vi "RT Driver VI.vi"(7 "Operation":T1, 11 "Device Reference in":T2 format="%.0x") -> (0 "Error Code":i32)   [LabVIEW 2019, in "Inline Telemetry Prototype Engine.lvlib"]
uses:
  Inline Telemetry Prototype Engine.lvlib
  <vilib>/NI VeriStand/Custom Device API/Custom Device Item Ref.ctl
  <vilib>/NI VeriStand/Custom Device API/Hardware Interface Driver VI Operation.ctl
  <vilib>/NI VeriStand/Custom Device API/Data Access Type.ctl
  Inline Async CD Template/Engine/Loop Data.ctl
  <vilib>/NI VeriStand/Custom Device API/Block Data Reference.ctl
  <vilib>/NI VeriStand/Custom Device API/Data Reference.ctl
  <vilib>/NI VeriStand/Custom Device API/Global Data Refs.vi
  <vilib>/NI VeriStand/Custom Device API/Custom Device API.lvlib
  Inline Async CD Template/Engine/Inline Async CD Template Engine.lvlib
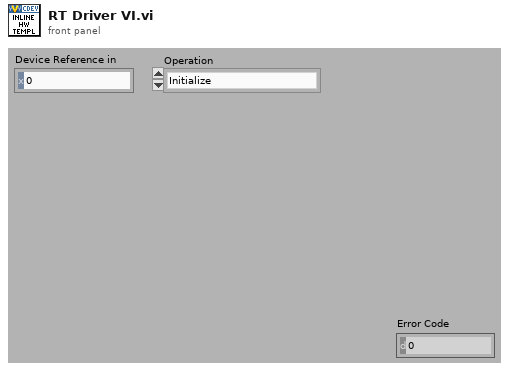
[diagram p1: front panel]
types:
  T1 = typedef "Custom Device API.lvlib/Hardware Interface Driver VI Operation.ctl" = enum16{"Initialize", "Start", "Read Data from HW", "Write Data to HW", "Close"}
  T2 = typedef "Custom Device API.lvlib/Custom Device Item Ref.ctl" = u64
  T3 = typedef "Inline Async CD Template Engine.lvlib/Loop Data.ctl" = cluster{"Device Error":errorcluster, "Data FIFO":refnum<k33>, "Block Data Refs":T4[], "Data":dbl[]}
  T4 = typedef "Custom Device API.lvlib/Block Data Reference.ctl" = cluster{"Data Reference":T5, "Offset":u64, "Length":u64}
  T5 = typedef "Custom Device API.lvlib/Data Reference.ctl" = i32
  T6 = typedef "Custom Device API.lvlib/Data Access Type.ctl" = enum16{"Read", "Write"}
  T7 = cluster{"read mode":enum16{"polling", "blocking"}, "write mode":enum16{"polling", "blocking"}}
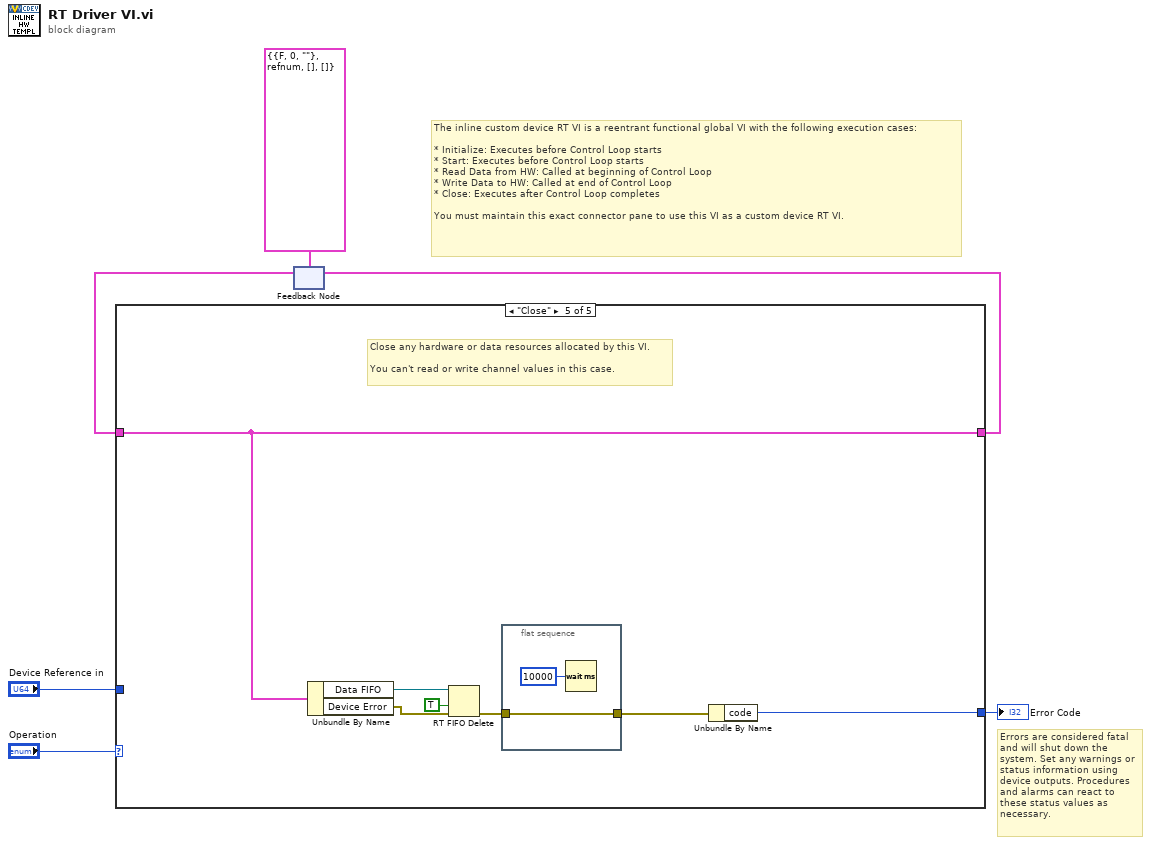
[diagram p0: block diagram]
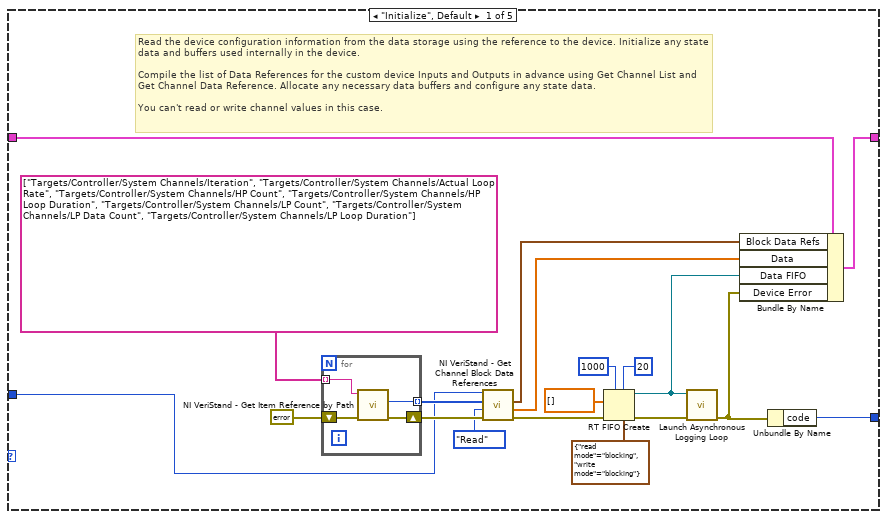
[diagram p2: hidden frame]
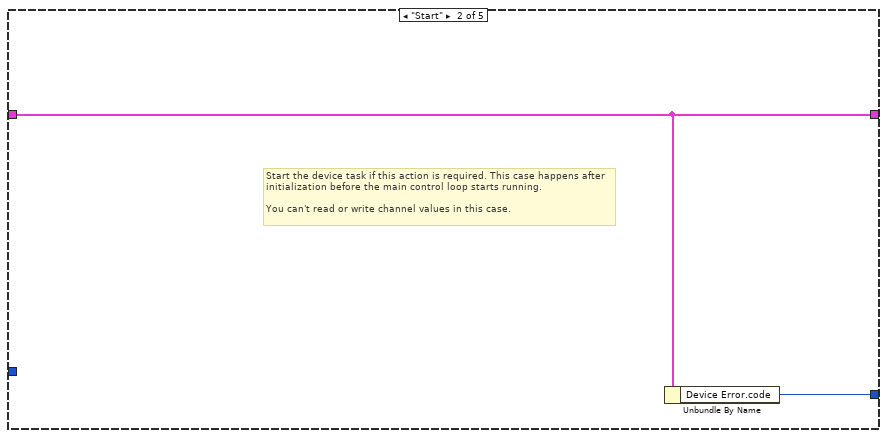
[diagram p3: hidden frame]
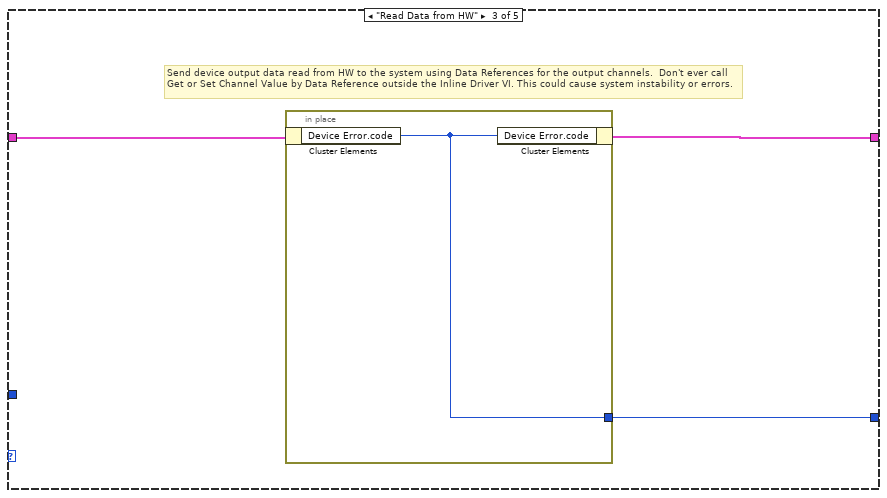
[diagram p4: hidden frame]
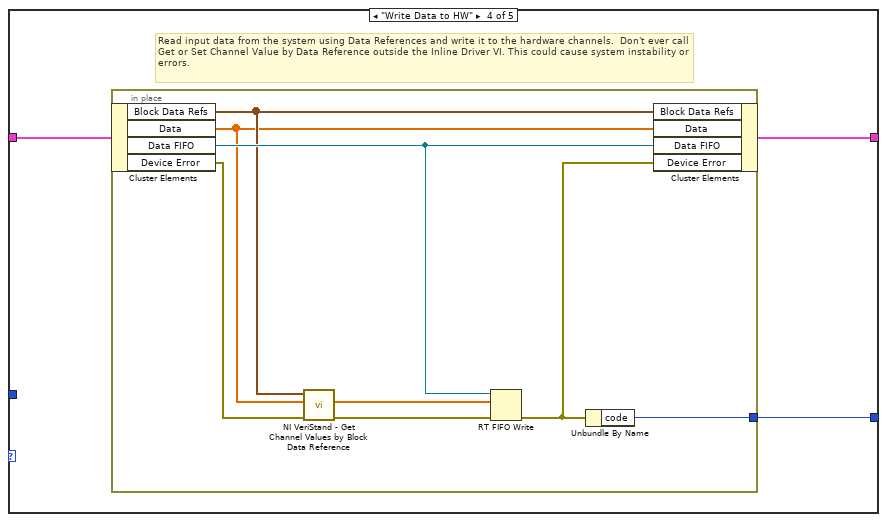
[diagram p5: hidden frame]
diagram:
  # "Errors are considered fatal and will shut down the system. Set any warnings or status information using device outputs. Procedures and alarms can react to these status values as necessary."
  # "The inline custom device RT VI is a reentrant functional global VI with the following execution cases:\n\n* Initialize: Executes before Control Loop starts\n* Start: Executes before Control Loop starts\n* Read Data from HW: Called at beginning of Control Loop\n* Write Data to HW: Called at end of Control Loop\n* Close: Executes after Control Loop completes\n\nYou must maintain this exact connector pane to use this VI as a custom device RT VI."
  n1 = feedback #1(T3 {"Device Error"={"status"=FALSE, "code"=0, "source"=""}, "Data FIFO"=refnum, "Block Data Refs"=[], "Data"=[]} ("cluster")) -> (w4:T3)
  n2 = case shown="\"Close\"" "Operation" {
    tunnel: [w11 w30 w33 w36 w49] -> w5
    tunnel: w4 -> [w13 w30 w34 w38 w49]
    tunnel: "Device Reference in" -> [w15 _ _ _ _]
    tunnel: [w25 w31 w32 w37 w53] -> w2
    frame "Initialize", Default {
      # "Read the device configuration information from the data storage using the reference to the device. Initialize any state data and buffers used internally in the device.\n\nCompile the list of Data References for the custom device Inputs and Outputs in advance using Get Channel List and Get Channel Data Reference. Allocate any necessary data buffers and configure any state data.\n\nYou can't read or write channel values in this case."
      n3 = for {
        tunnel: [w28] -> w19 mode=indexing
        shift-right: [w29] -> w17
        shift-left: errorcluster {"status"=FALSE, "code"=0, "source"=""} ("error out") -> [w27]
        tunnel: string[] ["Targets/Controller/System Channels/Iteration", "Targets/Controller/System Channels/Actual Loop Rate", "Targets/Controller/System Channels/HP Count", "Targets/Controller/System Channels/HP Loop Duration", "Targets/Controller/System Channels/LP Count", "Targets/Controller/System Channels/LP Data Count", "Targets/Controller/System Channels/LP Loop Duration"] -> [w26] mode=indexing
        n4 = call <vilib>:"NI VeriStand - Get Item Reference by Path.vi"("error in (no error)"=w27, "Item Path in"=w26) -> ("error out"=w29:errorcluster, "Item Ref"=w28:T2)  [unwired: 6 in, 2 out]
      }
      n5 = call <vilib>:"NI VeriStand - Get Channel Block Data References.vi"("error in (no error)"=w17, "Access"=Data_Access_Type."Read", "Channel Refs"=w19, "Device Ref in"=w15) -> ("error out"=w18:errorcluster, "Values Array"=w12:dbl[], "Block Data Refs"=w10:T4[])  [unwired: 4 in, 1 out]
      n6 = RT FIFO Create(1:dbl[] [], 3:w18, 4:u32 1000 ("size (10)"), 6:u32 20 ("elements in array (1)"), 7:T7 {"read mode"=enum."blocking", "write mode"=enum."blocking"} ("r/w modes (polling,polling)")) -> (8:w9:refnum<k33>, 11:w8:errorcluster)  [unwired: 3 in, 1 out]
      n7 = call "Launch Asynchronous Logging Loop.vi"("error in (no error)"=w8, "Log Data FIFO"=w9) -> ("error out"=w7:errorcluster)  [unwired: 9 in]
      n8 = Bundle By Name(cluster=w13, "Block Data Refs"=w10, "Data"=w12, "Data FIFO"=w9, "Device Error"=w7) -> (w11:T3)
      n9 = Unbundle By Name(w7) -> ("code"=w25:i32)
    }
    frame "Start" {
      # "Start the device task if this action is required. This case happens after initialization before the main control loop starts running.\n\nYou can't read or write channel values in this case."
      n10 = Unbundle By Name(w30) -> ("Device Error.code"=w31:i32)
    }
    frame "Read Data from HW" {
      # "Send device output data read from HW to the system using Data References for the output channels.  Don't ever call Get or Set Channel Value by Data Reference outside the Inline Driver VI. This could cause system instability or errors."
      n11 = in-place {
        in-place-border: [w35] -> w32
        n12 = in-place-cluster #2(w34) -> ("Device Error.code"=w35:i32)
        n13 = in-place-cluster #2("Device Error.code"=w35) -> (w33:T3)
      }
    }
    frame "Write Data to HW" {
      # "Read input data from the system using Data References and write it to the hardware channels.  Don't ever call Get or Set Channel Value by Data Reference outside the Inline Driver VI. This could cause system instability or errors."
      n14 = in-place {
        in-place-border: [w39] -> w37
        n15 = in-place-cluster #3(w38) -> ("Block Data Refs"=w42:T4[], "Data"=w41:dbl[], "Data FIFO"=w43:refnum<k33>, "Device Error"=w40:errorcluster)
        n16 = call <vilib>:"NI VeriStand - Get Channel Values by Block Data Reference.vi"("error in (no error)"=w40, "Values Array in"=w41, "Block Data Ref"=w42) -> ("error out"=w46:errorcluster, "Values Array out"=w45:dbl[])  [unwired: 6 in, 1 out]
        n17 = RT FIFO Write(0:w43, 1:w45, 3:w46) -> (11:w44:errorcluster)  [unwired: 2 in, 3 out]
        n18 = Unbundle By Name(w44) -> ("code"=w39:i32)
        n19 = in-place-cluster #3("Block Data Refs"=w42, "Data"=w41, "Data FIFO"=w43, "Device Error"=w44) -> (w36:T3)
      }
    }
    frame "Close" {
      # "Close any hardware or data resources allocated by this VI.\n\nYou can't read or write channel values in this case."
      n20 = Unbundle By Name(w49) -> ("Data FIFO"=w52:refnum<k33>, "Device Error"=w51:errorcluster)
      n21 = RT FIFO Delete(0:w52, 2:TRUE ("force destroy? (F)"), 3:w51) -> (11:w48:errorcluster)
      n22 = flat-sequence {
        tunnel: w48 -> [w54]
        tunnel: [w54] -> w47
        frame #0 {
          n23 = Wait (ms)(milliseconds to wait=u32 10000) -> ()  [unwired: 1 out]
        }
      }
      n24 = Unbundle By Name(w47) -> ("code"=w53:i32)
    }
  }
  "Error Code" <- w2
  n25 = feedback-in #1(w5) -> ()
